vi "test_libssh2_userauth_publickey_fromfile.vi"() -> ()   [LabVIEW 2017, in "integration_tests.lvlib"]
uses:
  integration_tests.lvlib
  libssh2/libssh2_session_handshake_tcp.vi
  libssh2/libssh2_init_default.vi
  libssh2/libssh2_session_init_ex.vi
  <vilib>/Utility/tcp.llb/TCP Get Raw Net Object.vi
  libssh2/libssh2_session_handshake_socket.vi
  libssh2/libssh2.lvlib
  support/support.lvlib
  <vilib>/PNR/Transparent Assertions/Transparent Assertions/Transparent Assertions.lvlib
panel:
  out "error out":errorcluster
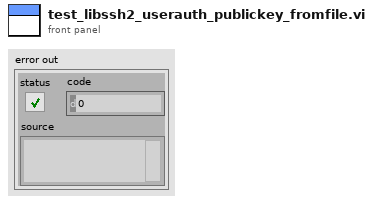
[diagram p1: front panel]
types:
  T1 = typedef "libssh2.lvlib/Session Refnum.ctl" = refnum<k1>
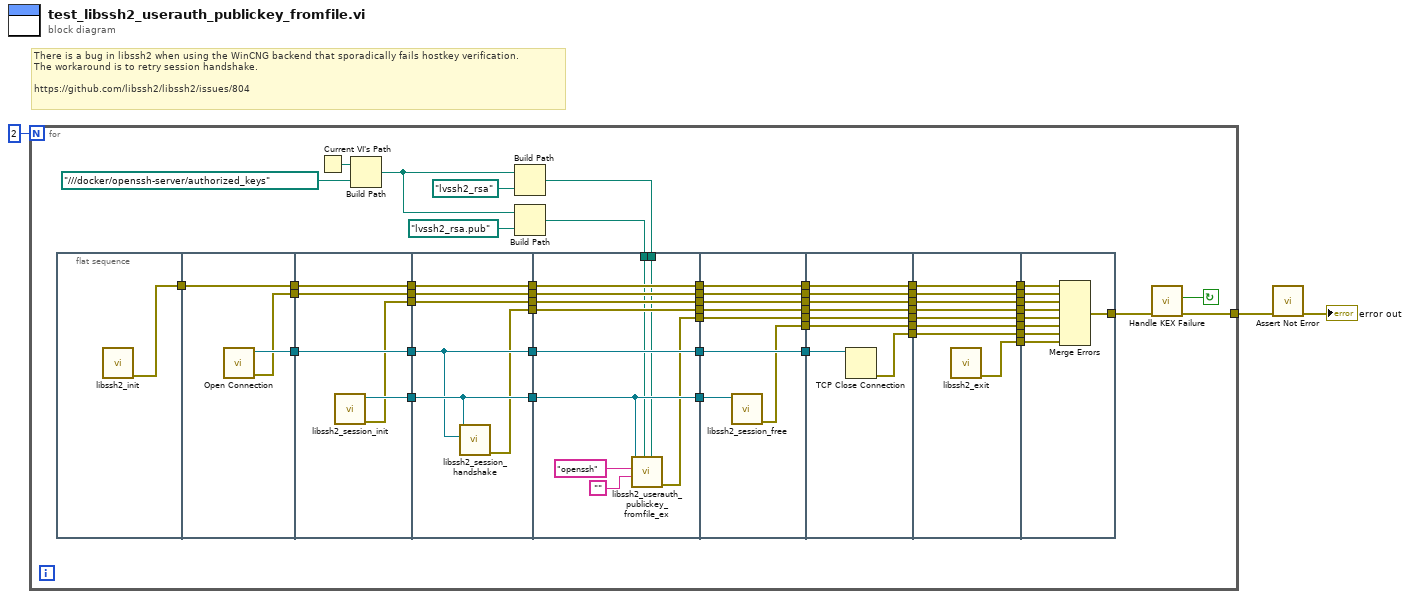
[diagram p0: block diagram]
diagram:
  # "There is a bug in libssh2 when using the WinCNG backend that sporadically fails hostkey verification.\nThe workaround is to retry session handshake.\n\nhttps://github.com/libssh2/libssh2/issues/804"
  n1 = for {
    N: 2 -> [_]
    tunnel: [w8] -> w2
    stop <- w9 continue-if-true
    n2 = flat-sequence {
      tunnel: [w58] -> w57
      tunnel: [w61] -> w56
      tunnel: w57 -> [w60]
      tunnel: [w60] -> w55
      tunnel: [w59] -> w54
      tunnel: w56 -> [w66]
      tunnel: [w66] -> w53
      tunnel: w55 -> [w65]
      tunnel: [w65] -> w52
      tunnel: w54 -> [w64]
      tunnel: [w64] -> w51
      tunnel: [w63] -> w50
      tunnel: [w62] -> w49
      tunnel: w53 -> [w68]
      tunnel: [w68] -> w48
      tunnel: w52 -> [w72]
      tunnel: [w72] -> w47
      tunnel: w51 -> [w71]
      tunnel: [w71] -> w46
      tunnel: [w70] -> w45
      tunnel: w50 -> [w70]
      tunnel: w49 -> [w69]
      tunnel: [w69] -> w44
      tunnel: [w67] -> w43
      tunnel: w48 -> [w83]
      tunnel: [w83] -> w42
      tunnel: w47 -> [w82]
      tunnel: [w82] -> w41
      tunnel: w46 -> [w81]
      tunnel: [w81] -> w40
      tunnel: w45 -> [w78]
      tunnel: w44 -> [w80]
      tunnel: [w80] -> w39
      tunnel: w43 -> [w79]
      tunnel: [w79] -> w38
      tunnel: [w78] -> w37
      tunnel: w13 -> [w75]
      tunnel: w12 -> [w74]
      tunnel: [w73] -> w7
      tunnel: w42 -> [w91]
      tunnel: [w91] -> w36
      tunnel: w41 -> [w90]
      tunnel: [w90] -> w35
      tunnel: w40 -> [w89]
      tunnel: [w89] -> w34
      tunnel: w39 -> [w88]
      tunnel: [w88] -> w33
      tunnel: w38 -> [w87]
      tunnel: [w87] -> w32
      tunnel: [w86] -> w31
      tunnel: w37 -> [w85]
      tunnel: w7 -> [w84]
      tunnel: [w84] -> w6
      tunnel: w36 -> [w99]
      tunnel: w35 -> [w98]
      tunnel: [w98] -> w30
      tunnel: w34 -> [w97]
      tunnel: [w97] -> w29
      tunnel: [w96] -> w28
      tunnel: w33 -> [w95]
      tunnel: [w95] -> w27
      tunnel: w32 -> [w94]
      tunnel: [w94] -> w26
      tunnel: [w93] -> w25
      tunnel: w31 -> [w93]
      tunnel: w6 -> [w92]
      tunnel: [w92] -> w5
      tunnel: w30 -> [w107]
      tunnel: [w107] -> w24
      tunnel: w29 -> [w106]
      tunnel: [w106] -> w23
      tunnel: w28 -> [w105]
      tunnel: [w105] -> w22
      tunnel: [w104] -> w21
      tunnel: w27 -> [w103]
      tunnel: [w103] -> w20
      tunnel: w26 -> [w102]
      tunnel: [w102] -> w19
      tunnel: [w101] -> w18
      tunnel: w25 -> [w101]
      tunnel: w5 -> [w100]
      tunnel: [w100] -> w4
      tunnel: w24 -> [w116]
      tunnel: w23 -> [w115]
      tunnel: w22 -> [w114]
      tunnel: w21 -> [w113]
      tunnel: w20 -> [w112]
      tunnel: w19 -> [w111]
      tunnel: w18 -> [w110]
      tunnel: [w109] -> w10
      tunnel: w4 -> [w108]
      frame #0 {
        n3 = call-poly "libssh2_init.vi"() -> ("error out"=w58:errorcluster)  [unwired: 11 in]
      }
      frame #1 {
        n4 = call "Open Connection.vi"() -> ("error out"=w59:errorcluster, "connection ID"=w61:refnum<k5>)  [unwired: 10 in]
      }
      frame #2 {
        n5 = call "libssh2_session_init.vi"() -> ("error out"=w62:errorcluster, "session"=w63:T1)  [unwired: 10 in]
      }
      frame #3 {
        n6 = call-poly "libssh2_session_handshake.vi"("tcp connection"=w68, "session"=w70) -> ("error out"=w67:errorcluster)  [unwired: 9 in]
      }
      frame #4 {
        n7 = call "libssh2_userauth_publickey_fromfile_ex.vi"("private key"=w74, "public key"=w75, "passphrase"="", "username"="openssh", "session"=w78) -> ("error out"=w73:errorcluster)  [unwired: 6 in]
      }
      frame #5 {
        n8 = call "libssh2_session_free.vi"("session"=w85) -> ("error out"=w86:errorcluster)  [unwired: 10 in]
      }
      frame #6 {
        n9 = TCP Close Connection(connection ID=w99) -> (error out=w96:errorcluster)  [unwired: 2 in, 1 out]
      }
      frame #7 {
        n10 = call "libssh2_exit.vi"() -> ("error out"=w104:errorcluster)  [unwired: 11 in]
      }
      frame #8 {
        n11 = Merge Errors(w116, w115, w112, w111, w108, w110, w114, w113) -> (w109:errorcluster)
      }
    }
    n12 = Current VI's Path() -> (path=w11:path)
    n13 = Build Path(base path=w11, name or relative path=path "../../../docker/openssh-server/authorized_keys" ("stripped path")) -> (appended path=w14:path)
    n14 = Build Path(base path=w14, name or relative path=path "lvssh2_rsa" ("stripped path")) -> (appended path=w12:path)
    n15 = Build Path(base path=w14, name or relative path=path "lvssh2_rsa.pub" ("stripped path")) -> (appended path=w13:path)
    n16 = call "Handle KEX Failure.vi"("error in (no error)"=w10) -> ("error out"=w8:errorcluster, "KEX Failure"=w9:bool)  [unwired: 9 in]
  }
  n17 = call <vilib>:"Assert Not Error.vi"("error in (no error)"=w2) -> ("error out"=→"error out":errorcluster)  [unwired: 10 in]
